vi "Add E&S message to Text file.vi"(0 "refnum in":refnum<file>, 7 "E&S Message":T1={"Type"=enum."Error/Warning", "Originate time"=nan, "System"=0, "Loop"=9999, "Sub ID"=0, "Elevated priority"=FALSE, "E&S Message content"=variant}, 11 "error in (no error)":errorcluster, 12 "Simple(F)":bool) -> (4 "refnum out":refnum<file>, 15 "error out":errorcluster)   [LabVIEW 2011]
uses:
  emi Lib/System 01/0 - General/S&E reporting/Private/_emi_ S&E Message.ctl
  emi Lib/System 01/0 - General/S&E reporting/Private/_emi_ S&E Message type.ctl
  String outpyt type.ctl
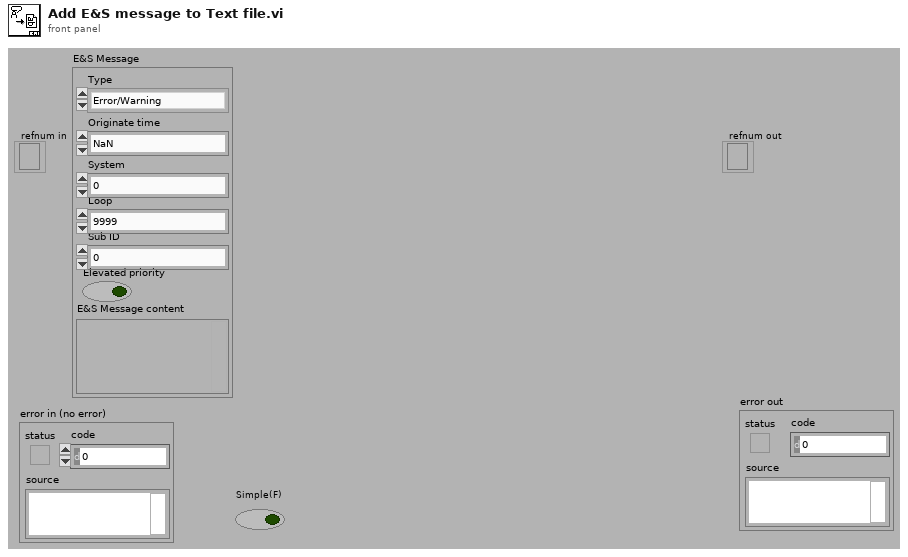
[diagram p1: front panel]
types:
  T1 = typedef "_emi_ S&E Message.ctl" = cluster{"Type":T2, "Originate time":dbl, "System":u8, "Loop":u16, "Sub ID":u16, "Elevated priority":bool, "E&S Message content":variant}
  T2 = typedef "_emi_ S&E Message type.ctl" = enum16{"Error/Warning", "Note", "Debug", "Event", "Alarm Analog", "Alarm Digital", "Annotation"}
  T3 = typedef "String outpyt type.ctl" = enum16{"Full File hist", "Simple File hist", "Displ Hist one type", "Displ Hist mult types", "Displ Stat one type", "Displ Stat Mult type"}
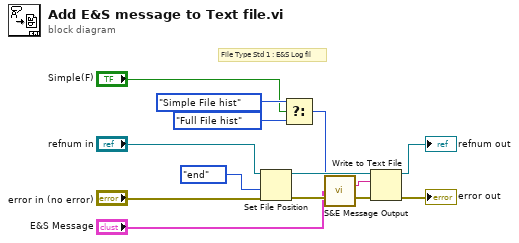
[diagram p0: block diagram]
diagram:
  # "File Type Std 1 : E&S Log fil"
  n1 = Set File Position(refnum="refnum in", from (0:start)=enum16{"start", "end", "current"}."end", error in="error in (no error)") -> (refnum out=w9:refnum<file>, error out=w8:errorcluster)  [unwired: 1 in]
  n2 = Select(t=String_outpyt_type."Simple File hist" ("Type(File Hist)"), s="Simple(F)", f=String_outpyt_type."Full File hist" ("Type(File Hist)")) -> (s? t:f=w5:T3)
  n3 = call "S&E Message Output.vi"("Type(File Hist)"=w5, "E&S Message"="E&S Message", "error in (no error)"=w8) -> ("String(File)"=w2:string, "error out"=w7:errorcluster)  [unwired: 10 in, 1 out]
  n4 = Write to Text File(file (use dialog)=w9, text=w2, error in=w7) -> (refnum out=→"refnum out":refnum<file>, error out=→"error out":errorcluster)  [unwired: 1 in, 1 out]
